vi "Copy Config to All Projects.vi"(8 "error in (no error)":errorcluster, 11 "Workspace dir":path) -> (0 "error out":errorcluster)   [LabVIEW 2010]
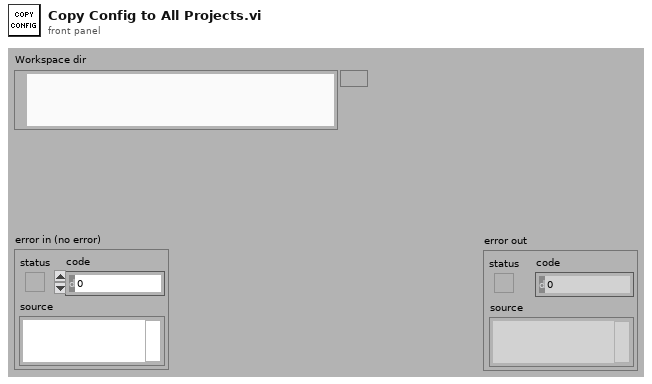
[diagram p1: front panel]
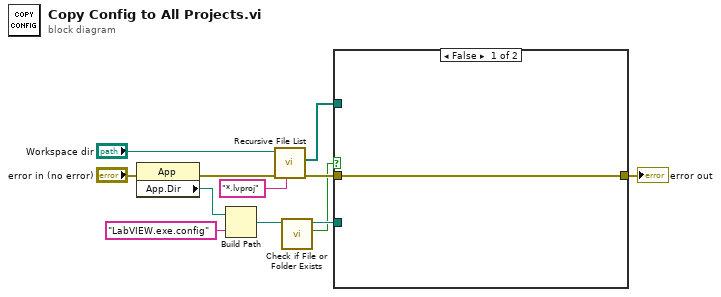
[diagram p0: block diagram]
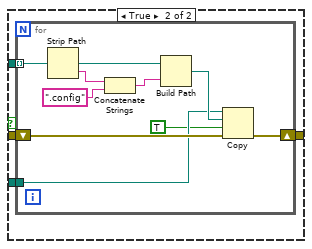
[diagram p2: hidden frame]
diagram:
  n1 = property class="App"(error in="error in (no error)") -> (error out=w6:errorcluster, "App.Dir"=w8:path)  [unwired: 1 in, 1 out]
  n2 = Build Path(base path=w8, name or relative path="LabVIEW.exe.config") -> (appended path=w5:path)
  n3 = call <vilib>:"Recursive File List.vi"("pattern"="*.lvproj", "error in (no error)"=w6, "Folder Path"="Workspace dir") -> ("error out"=w10:errorcluster, "All Files in Dir"=w9:path[])  [unwired: 4 in, 3 out]
  n4 = call <vilib>:"Check if File or Folder Exists.vi"("path"=w5) -> ("file or folder exists?"=w1:bool, "dup path"=w2:path)  [unwired: 8 in, 1 out]
  n5 = case shown="False" w1 {
    tunnel: w10 -> [w13 w17]
    tunnel: w9 -> [_ w16]
    tunnel: [w13 w15] -> w3
    tunnel: w2 -> [_ w14]
    frame False {
    }
    frame True {
      n6 = for {
        shift-right: [w18] -> w15
        shift-left: w17 -> [w22]
        tunnel: w16 -> [w27] mode=indexing
        tunnel: w14 -> [w20]
        n7 = Strip Path(path=w27) -> (stripped path=w26:path, name=w25:string)
        n8 = Concatenate Strings(w25, ".config" ("string")) -> (w23:string)
        n9 = Build Path(base path=w26, name or relative path=w23) -> (appended path=w21:path)
        n10 = Copy(8:w22, 9:TRUE ("overwrite (F)"), 10:w21, 11:w20) -> (0:w18:errorcluster)  [unwired: 1 in, 2 out]
      }
    }
  }
  "error out" <- w3
